vi "DWDT Waveform Duration.vi"(7 "open interval? (T)":bool=TRUE caption="开区间？(T)", 8 "error in (no error)":errorcluster caption="错误输入（无错误）", 11 "waveform in":digitalwaveform(waveform)={"t0"=timestamp(0 s since 1904-01-01), "dt"=0.0, "Y"={"transitions"=[], "data"=[]}, "error"={"status"=FALSE, "code"=37421928, "source"=""}} caption="波形输入") -> (0 "error out":errorcluster caption="错误输出", 2 "duration":dbl caption="持续时间" format="%0.2f", 3 "waveform out":digitalwaveform(waveform)={"t0"=timestamp(0 s since 1904-01-01), "dt"=0.0, "Y"={"transitions"=[], "data"=[]}, "error"={"status"=FALSE, "code"=37421928, "source"=""}} caption="波形输出")   [LabVIEW 2018]
doc: "使用下列公式计算<B>波形输入</B>的<B>持续时间</B>：<B>持续时间</B> = (采样数-1) x dx 通过连线数据至<B>波形输入</B>输入端可确定要使用的多态实例，也可手动选择实例。"
panel:
  in  "Empty Waveform":digitalwaveform(waveform)={"t0"=timestamp(0 s since 1904-01-01), "dt"=0.0, "Y"={"transitions"=[], "data"=[]}, "error"={"status"=FALSE, "code"=37421928, "source"=""}} caption="空波形"
  # "开"
  # "闭"
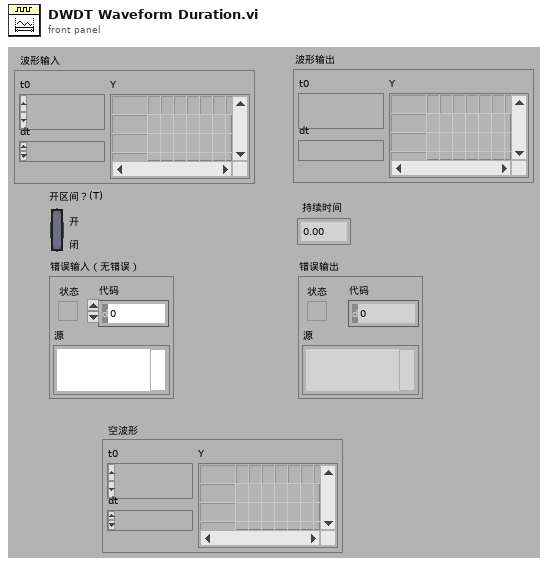
[diagram p1: front panel]
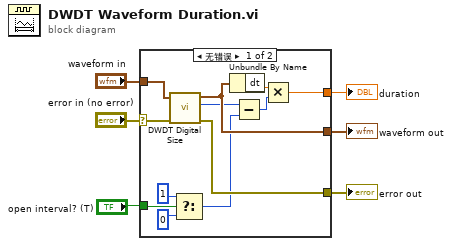
[diagram p0: block diagram]
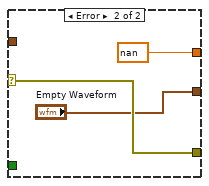
[diagram p2: hidden frame]
diagram:
  n1 = case shown="无错误" "error in (no error)" {
    selector: "error in (no error)" -> [w17 w20]
    tunnel: "waveform in" -> [w15 _]
    tunnel: [w18 nan] -> w6
    tunnel: [w14 "Empty Waveform"] -> w5
    tunnel: [w16 w20] -> w3
    tunnel: "open interval? (T)" -> [w12 _]
    frame No Error {
      n2 = call "DWDT Digital Size.vi"("error in (no error)"=w17, "digital waveform in"=w15) -> ("error out"=w16:errorcluster, "number of samples"=w9:i32, "digital waveform out"=w14:digitalwaveform)  [unwired: 6 in, 1 out]
      n3 = Select(t=1 ("number of samples"), s=w12, f=0 ("number of samples")) -> (s? t:f=w7:i32)
      n4 = Unbundle By Name(w14) -> ("dt"=w13:dbl)
      n5 = Subtract(x=w9, y=w7) -> (x-y=w8:i32)
      n6 = Multiply(x=w13, y=w8) -> (x*y=w18:dbl)
    }
    frame Error {
      # "Incoming Error"
    }
  }
  "duration" <- w6
  "waveform out" <- w5
  "error out" <- w3
